vi "Construct Listbox Bus Monitor.vi"(10 "Show Panel Boolean Name":string) -> (3 "ListboxBusMonitor out":refnum<class "ListboxBusMonitor.lvclass">)   [LabVIEW 2019, in "ListboxBusMonitor.lvlib" / "ListboxBusMonitor.lvclass"]
uses:
  <vilib>/gpm_packages/@cs/BusMonitor/ListboxBusMonitor/ListboxBusMonitor/ListboxBusMonitor.lvclass
  <vilib>/gpm_packages/@cs/BusMonitor/ListboxBusMonitor/ListboxBusMonitor/ListboxBusMonitor.lvclass/ListboxBusMonitor.ctl
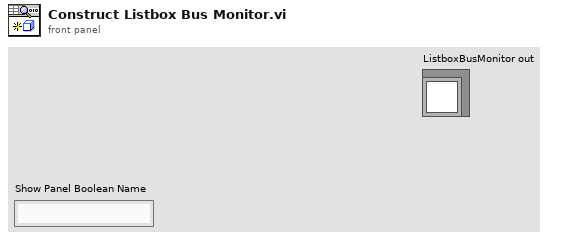
[diagram p1: front panel]
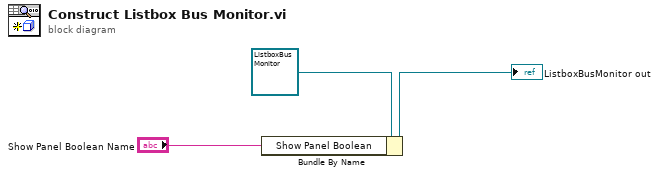
[diagram p0: block diagram]
diagram:
  n1 = Bundle By Name(cluster=refnum<class "ListboxBusMonitor.lvclass"> refnum ("ListboxBusMonitor in"), "Show Panel Boolean"="Show Panel Boolean Name") -> (→"ListboxBusMonitor out":refnum<class "ListboxBusMonitor.lvclass">)
